vi "NistTime2TS.vi"(1 "NIST Time":dbl format="%#_13g") -> (0 "Time Stamp":timestamp)   [LabVIEW 2014]
uses:
  <vilib>/Utility/miscctls.llb/LVDateTimeRec.ctl
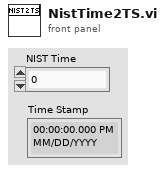
[diagram p1: front panel]
types:
  T1 = typedef "LVDateTimeRec.ctl" = cluster{"fractional second":dbl, "second":i32, "minute":i32, "hour":i32, "day of month":i32, "month":i32, "year":i32, "day of week":i32, "day of year":i32, "DST":i32}
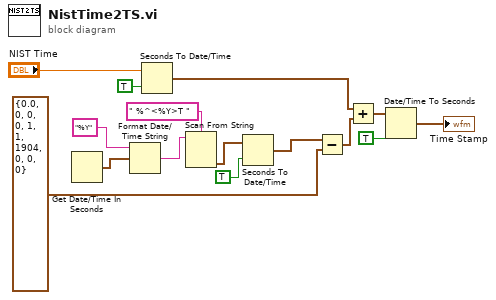
[diagram p0: block diagram]
diagram:
  n1 = Get Date/Time In Seconds() -> (seconds since 1Jan1904=w15:timestamp)
  n2 = Format Date/Time String(time format string (%c)="%Y", seconds (now)=w15) -> (date/time string=w14:string)  [unwired: 1 in]
  n3 = Seconds To Date/Time(time stamp (now)="NIST Time", to UTC (F)=TRUE) -> (date time rec=w4:T1)
  n4 = Scan From String(format string=" %^<%Y>T ", input string=w14) -> (output 1=w11:timestamp)  [unwired: 3 in, 3 out]
  n5 = Seconds To Date/Time(time stamp (now)=w11, to UTC (F)=TRUE) -> (date time rec=w9:T1)
  n6 = Subtract(x=w9, y=T1 {"fractional second"=0.0, "second"=0, "minute"=0, "hour"=0, "day of month"=1, "month"=1, "year"=1904, "day of week"=0, "day of year"=0, "DST"=0}) -> (x-y=w5:T1)
  n7 = Add(x=w4, y=w5) -> (x+y=w2:T1)
  n8 = Date/Time To Seconds(1:TRUE ("is UTC (F)"), 2:w2) -> (0:→"Time Stamp":timestamp)
